vi "Compare_Convert_Distance_to_Flywheel_Velocity.vi"() -> ()   [LabVIEW 2019]
panel:
  out "distance":dbl
  out "velocity":dbl
  in  "angle":dbl=30.0
  in  "terminal height":dbl=90.5
  out "Numeric":i32
  out "velocities":dbl[](array[numeric])
  out "distances":dbl[](array[numeric])
  out "Test Plot":cluster{dbl[], dbl[]}[](graph)
  in  "StopValue":dbl=300.0
  in  "StartValue":dbl
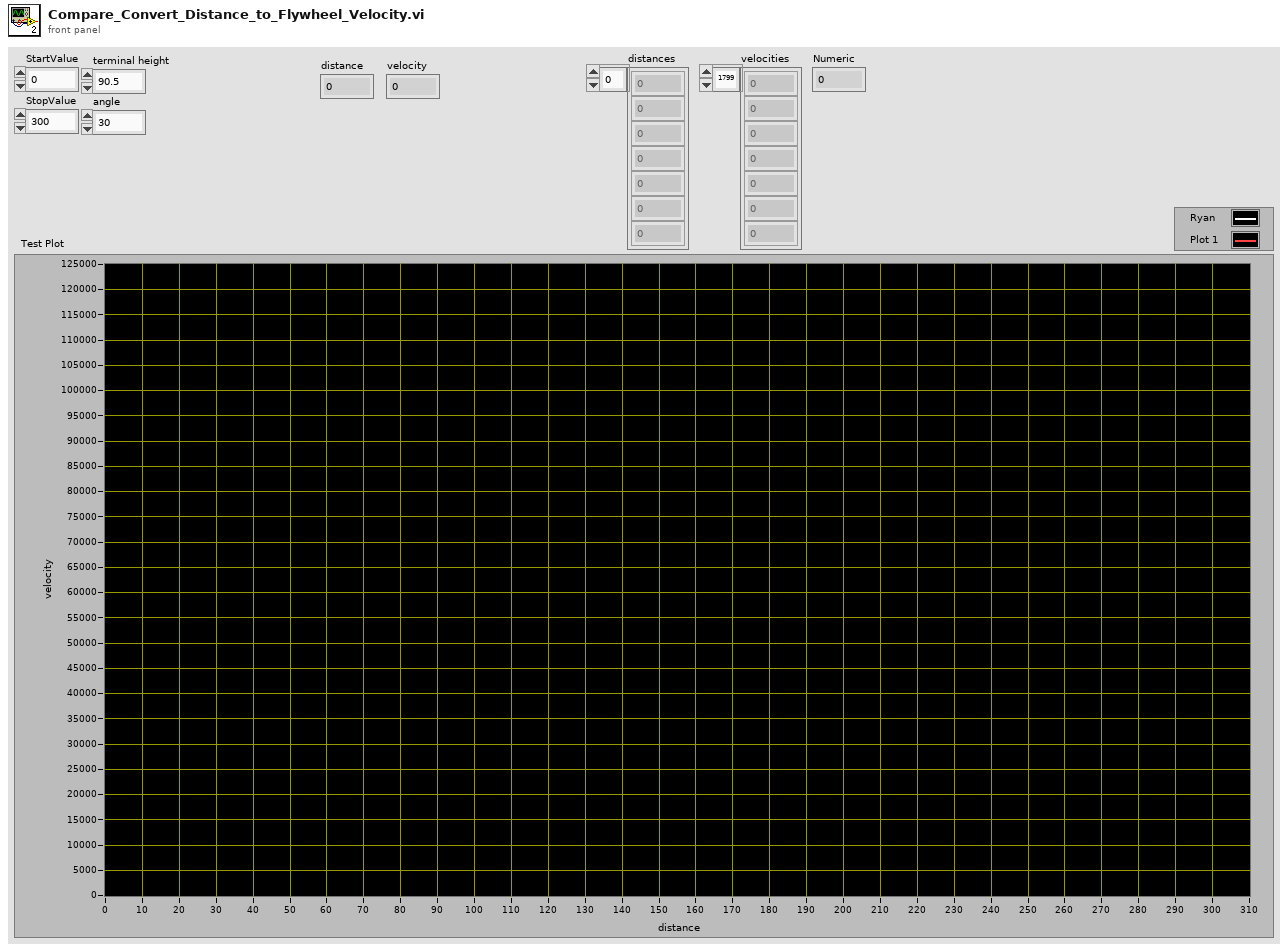
[diagram p1: front panel]
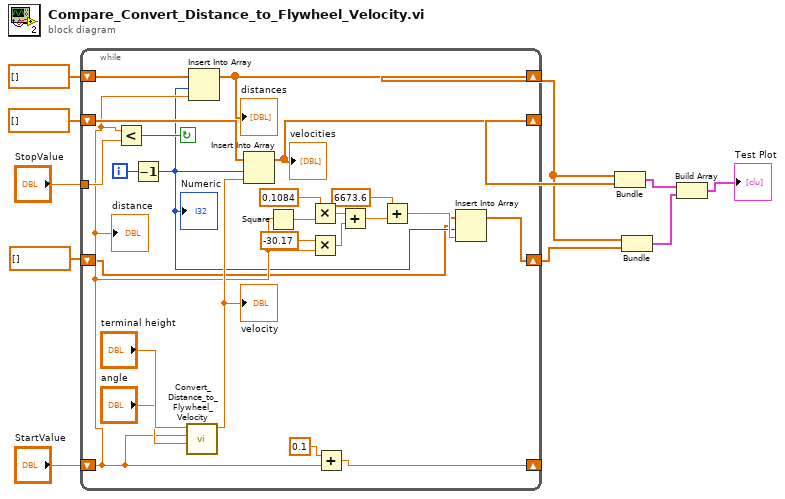
[diagram p0: block diagram]
diagram:
  n1 = while {
    shift-right: [w34] -> _
    shift-left: "StartValue" -> [w20]
    tunnel: "StopValue" -> [w33]
    shift-right: [w28] -> w5
    shift-left: dbl[] [] -> [w30]
    shift-right: [w27] -> w7
    shift-left: dbl[] [] -> [w29]
    shift-right: [w12] -> w4
    shift-left: dbl[] [] -> [w13]
    i -> [w31]
    stop <- w32 continue-if-true
    n2 = Less?(x=w20, y=w33) -> (x < y?=w32:bool)
    n3 = Decrement(x=w31) -> (x-1=w14:i32)
    "Numeric" <- w14
    n4 = call "Convert_Distance_to_Flywheel_Velocity.vi"("angle"="angle", "distance"=w20, "terminal height"="terminal height") -> ("velocity"=w24:dbl)  [unwired: 8 in]
    "velocity" <- w24
    n5 = Insert Into Array(array=w30, index=w14, new element=w20) -> (w28:dbl[])
    "distances" <- w28
    n6 = Insert Into Array(array=w29, index=w14, new element=w24) -> (w27:dbl[])
    "velocities" <- w27
    n7 = Square(x=w20) -> (x^2=w23:dbl)
    n8 = Multiply(x=0.1084, y=w23) -> (x*y=w21:dbl)
    n9 = Multiply(x=-30.17, y=w20) -> (x*y=w18:dbl)
    n10 = Add(x=0.1, y=w20) -> (x+y=w34:dbl)
    n11 = Add(x=w21, y=w18) -> (x+y=w17:dbl)
    n12 = Add(x=6673.6, y=w17) -> (x+y=w15:dbl)
    n13 = Insert Into Array(array=w13, index=w14, new element=w15) -> (w12:dbl[])
    "distance" <- w20
  }
  n14 = Bundle(w5, w7) -> (w3:cluster{dbl[], dbl[]})  [unwired: 1 in]
  n15 = Bundle(w5, w4) -> (w2:cluster{dbl[], dbl[]})  [unwired: 1 in]
  n16 = Build Array(w3, w2) -> (→"Test Plot":cluster{dbl[], dbl[]}[])
